vi "setUserEvents.vi"(10 "UserEvents":T1, 11 "UserEvents in":refnum<class "UserEvents.lvclass">) -> (3 "UserEvents out":refnum<class "UserEvents.lvclass">)   [LabVIEW 2016, in "UserEvents.lvclass"]
uses:
  UserEvents.lvclass
  Types/UserEvents.ctl
  Communicator/Topics/EventSummaryState.ctl
  Types/Timestamp.ctl
  Types/SummaryStates.ctl
  Types/ProcessCommandEvent.ctl
  Commands/Command/Command.lvclass
  Types/ShutdownEvent.ctl
  Communicator/Topics/CommandId.ctl
  Communicator/Topics/TelemetryFPGAData.ctl
  UserEvents.lvclass/UserEvents.ctl
  Types/M1M3SupportTypes.lvlib
  Communicator/M1M3Communicator.lvlib
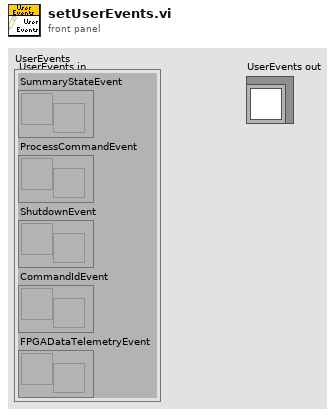
[diagram p1: front panel]
types:
  T1 = typedef "M1M3SupportTypes.lvlib/UserEvents.ctl" = cluster{"SummaryStateEvent":refnum<user-event>, "ProcessCommandEvent":refnum<user-event>, "ShutdownEvent":refnum<user-event>, "CommandIdEvent":refnum<user-event>, "FPGADataTelemetryEvent":refnum<user-event>}
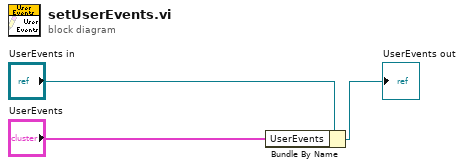
[diagram p0: block diagram]
diagram:
  n1 = Bundle By Name(cluster="UserEvents in", "UserEvents"="UserEvents") -> (→"UserEvents out":refnum<class "UserEvents.lvclass">)
